vi "ActionVIOnLoad.vi"(8 "error in (no error)":errorcluster, 11 "Device Item Ref in":T1 format="%.0x") -> (0 "error out":errorcluster, 3 "Device Item Ref out":T1 format="%.0x")   [LabVIEW 2019, in "J1939 Addon System Explorer.lvlib"]
uses:
  J1939 Addon System Explorer.lvlib
  <vilib>/NI VeriStand/Custom Device API/Custom Device Item Ref.ctl
  <vilib>/NI VeriStand/Custom Device API/Custom Device Channel.ctl
  <vilib>/NI VeriStand/Custom Device API/Custom Device Channel Type.ctl
  NationalInstruments.VeriStand.SystemDefinitionAPI
  Addon Shared/SubVIs/Constants.vi
  <vilib>/NI/NI VeriStand Advanced SysDef API/_SubVIs/SysDef.Search.GUIDs.vi
  <vilib>/NI/NI VeriStand Advanced SysDef API/_SubVIs/SysDef.Search.Parent.vi
  Addon Shared/J1939 Addon Shared.lvlib
  <vilib>/NI/NI VeriStand Advanced SysDef API/SysDef API/Advanced System Definition.lvlib
  <vilib>/NI VeriStand/Custom Device API/Custom Device API.lvlib
  SubModules/Frame-Protection-Support/Source/System Explorer/Protection and Counter Support System Explorer.lvlib
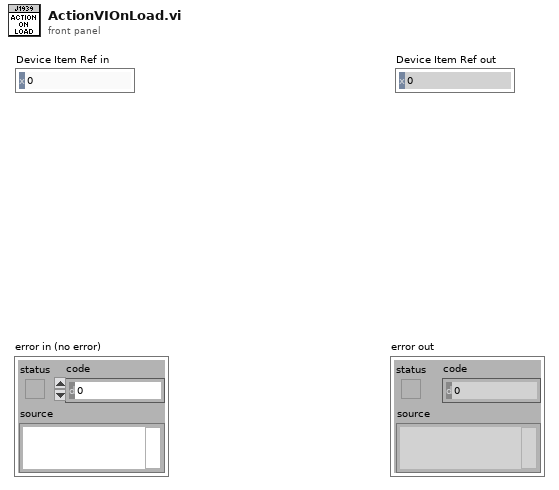
[diagram p1: front panel]
types:
  T1 = typedef "Custom Device API.lvlib/Custom Device Item Ref.ctl" = u64
  T2 = typedef "Custom Device API.lvlib/Custom Device Channel.ctl" = cluster{"Type":T3, "Units":string, "Default Value":dbl, "Faultable":bool, "Scalable":bool}
  T3 = typedef "Custom Device API.lvlib/Custom Device Channel Type.ctl" = enum16{"Input", "Output"}
  T4 = typedef "Protection and Counter Support System Explorer.lvlib/Protection Signal Settings.ctl" = cluster{"Input Channels":T5[], "Protection Type":T6}
  T5 = typedef "Protection and Counter Support System Explorer.lvlib/Protection Signal Linked Channel.ctl" = cluster{"Node Ref":T1}
  T6 = typedef "Protection and Counter Support Shared.lvlib/Protection Type.ctl" = enum16{"Arb ID + Bytes Checksum with Inversion", "Arb ID + Bytes CRC with Inversion", "Reversed Raw Signal Checksum with Inversion", "Concatenated Two's Compliment"}
  T7 = typedef "Advanced System Definition.lvlib/TreeItem.Info.ctl" = cluster{"Name":string, "Description":string, "GUID":string, "Is Channel":bool, "Channel":T2, "Is Waveform":bool, "Waveform":T8}
  T8 = typedef "Custom Device API.lvlib/Custom Device Waveform.ctl" = cluster{"Data Type":T9, "Units":string}
  T9 = typedef "Custom Device API.lvlib/Custom Device Waveform DataType.ctl" = enum16{"Double", "Complex Double"}
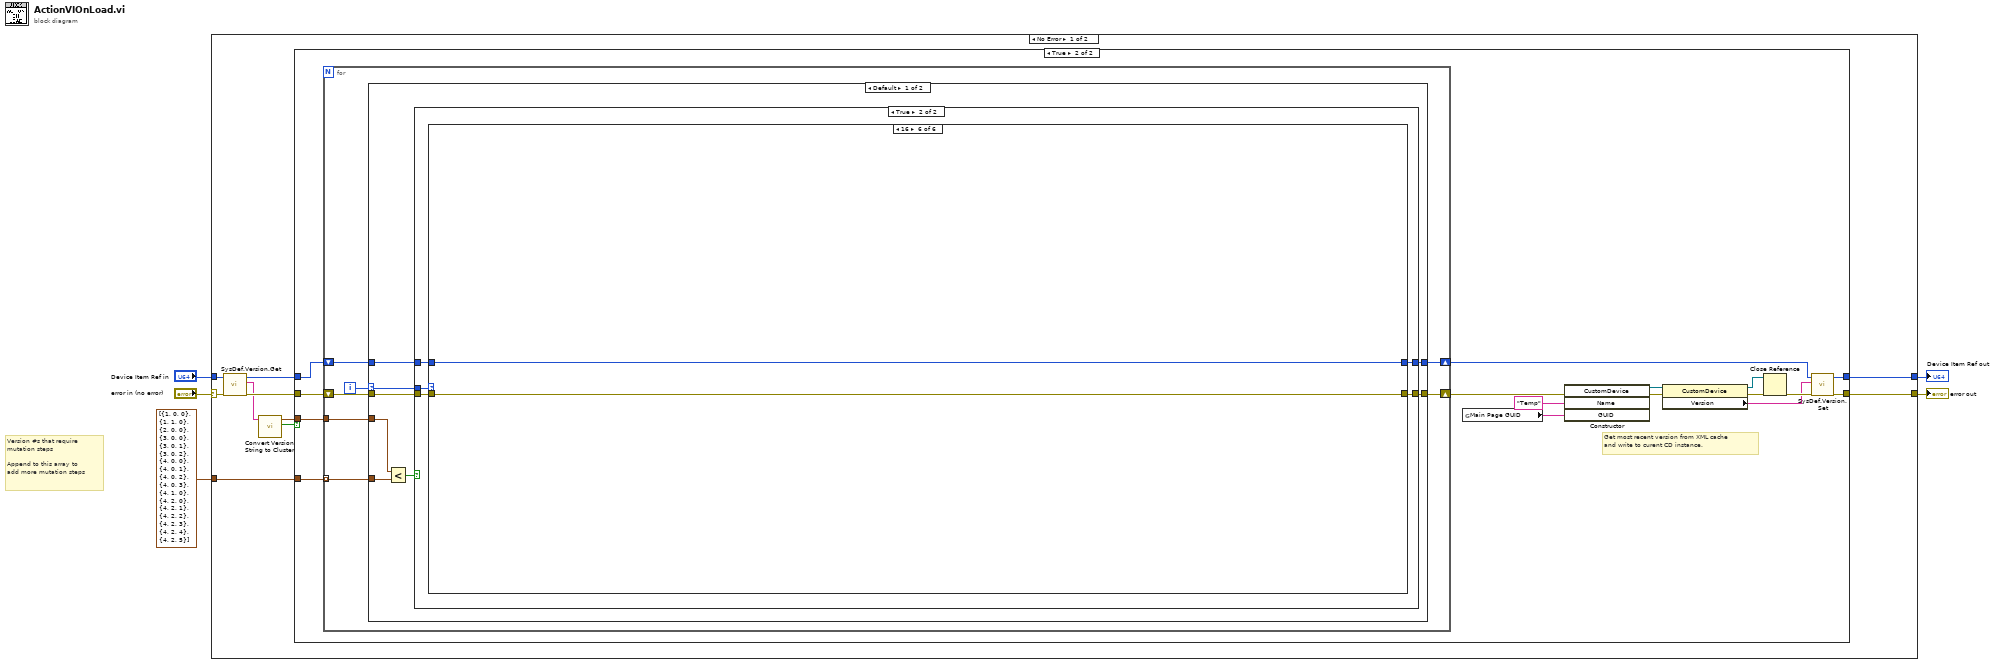
[diagram p0: block diagram]
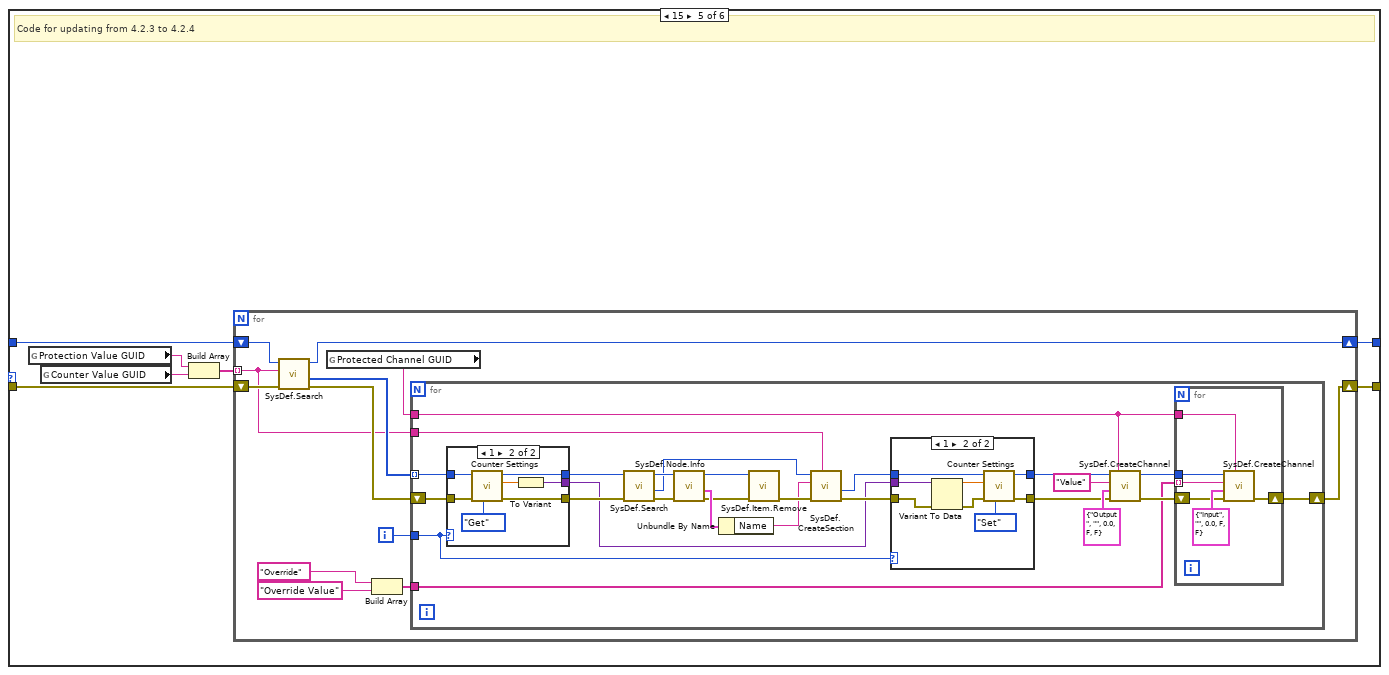
[diagram p8: hidden frame]
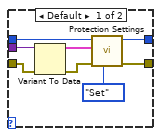
[diagram p9: hidden frame]
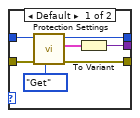
[diagram p10: hidden frame]
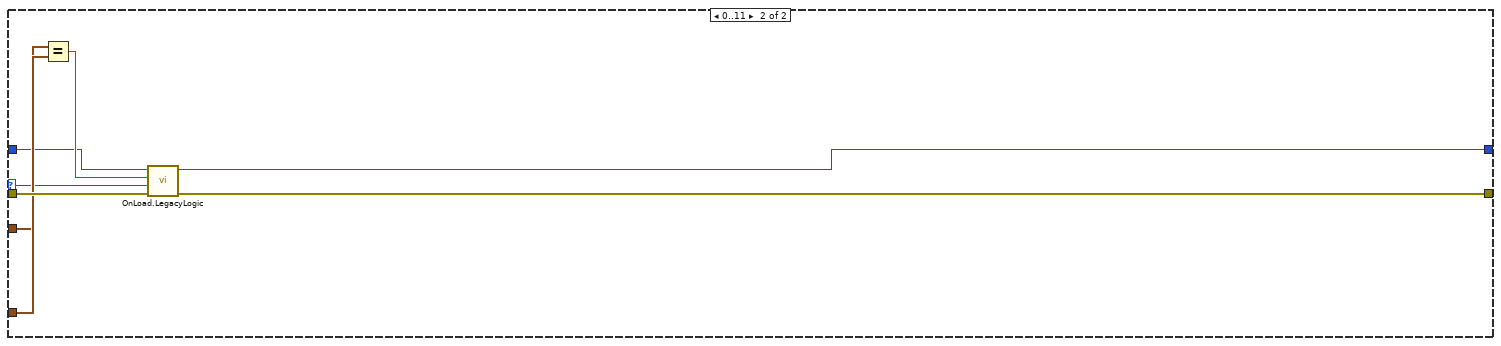
[diagram p11: hidden frame]
diagram:
  # "Version #s that require\nmutation steps\n\nAppend to this array to\nadd more mutation steps"
  n1 = case shown="No Error" "error in (no error)" {
    selector: "error in (no error)" -> [w12 w156]
    tunnel: [w14 w156] -> w1
    tunnel: "Device Item Ref in" -> [w11 w155]
    tunnel: [w13 w155] -> w2
    tunnel: cluster{i32, i32, i32}[] [{1, 0, 0}, {1, 1, 0}, {2, 0, 0}, {3, 0, 0}, {3, 0, 1}, {3, 0, 2}, {4, 0, 0}, {4, 0, 1}, {4, 0, 2}, {4, 0, 3}, {4, 1, 0}, {4, 2, 0}, {4, 2, 1}, {4, 2, 2}, {4, 2, 3}, {4, 2, 4}, {4, 2, 5}] -> [w15 _]
    frame No Error {
      n2 = call <vilib>:"SysDef.Version.Get.vi"("error in (no error)"=w12, "nodeID"=w11) -> ("error out"=w10:errorcluster, "Version"=w8:string, "nodeID out"=w9:u64)  [unwired: 7 in]
      n3 = call "Convert Version String to Cluster.vi"("Version"=w8) -> ("Version Valid?"=w6:bool, "Version"=w7:cluster{i32, i32, i32})  [unwired: 9 in]
      n4 = case shown="True" w6 {
        tunnel: w15 -> [_ w33]
        tunnel: [w17 w26] -> w14
        tunnel: [w16 w25] -> w13
        tunnel: w10 -> [w17 w22]
        tunnel: w9 -> [w16 w21]
        tunnel: w7 -> [_ w18]
        frame False {
        }
        frame True {
          # "Get most recent version from XML cache\nand write to curent CD instance."
          n5 = for {
            tunnel: w33 -> [w40] mode=indexing
            tunnel: w18 -> [w37]
            shift-right: [w35] -> w20
            shift-left: w21 -> [w36]
            shift-right: [w34] -> w19
            shift-left: w22 -> [w38]
            i -> [w39]
            n6 = case shown="Default" w39 {
              selector: w39 -> [w46 w149]
              tunnel: w38 -> [w44 w154]
              tunnel: [w42 w153] -> w34
              tunnel: w36 -> [w43 w147]
              tunnel: [w41 w152] -> w35
              tunnel: w40 -> [w48 w151]
              tunnel: w37 -> [w47 w150]
              frame Default {
                n7 = Less?(x=w47, y=w48) -> (x < y?=w45:bool)
                n8 = case shown="True" w45 {
                  tunnel: w46 -> [_ w55]
                  tunnel: w44 -> [w50 w54]
                  tunnel: w43 -> [w49 w53]
                  tunnel: [w50 w52] -> w42
                  tunnel: [w49 w51] -> w41
                  frame False {
                  }
                  frame True {
                    n9 = case shown="16" w55 {
                      tunnel: w54 -> [w57 w59 w61 w63 w69 w146]
                      tunnel: w53 -> [w56 w58 w60 w62 w66 w145]
                      tunnel: [w57 w59 w61 w63 w68 w146] -> w52
                      tunnel: [w56 w58 w60 w62 w67 w145] -> w51
                      frame 0..11, Default {
                        # "Previous on load scheme. Ignore."
                      }
                      frame 12 {
                        # "Code for updating from 4.2.0 to 4.2.1"
                      }
                      frame 13 {
                        # "Code for updating from 4.2.1 to 4.2.2"
                      }
                      frame 14 {
                        # "Code for updating from 4.2.2 to 4.2.3"
                      }
                      frame 15 {
                        # "Code for updating from 4.2.3 to 4.2.4"
                        n10 = global read "Constants.vi" "Protection Value GUID"() -> (w64:string)
                        n11 = global read "Constants.vi" "Counter Value GUID"() -> (w65:string)
                        n12 = Build Array(w64, w65) -> (w70:string[])
                        n13 = for {
                          shift-right: [w82] -> w67
                          shift-left: w66 -> [w81]
                          shift-right: [w77] -> w68
                          shift-left: w69 -> [w80]
                          tunnel: w70 -> [w73] mode=indexing
                          i -> [w72]
                          n14 = call-poly <vilib>:"SysDef.Search.vi"("error in (no error)"=w80, "GUID"=w73, "nodeID"=w81) -> ("error out"=w78:errorcluster, "Values Out"=w79:u64[], "nodeID out"=w82:u64)  [unwired: 5 in, 1 out]
                          n15 = global read "Constants.vi" "Protected Channel GUID"() -> (w71:string)
                          n16 = Build Array("Override" ("Override Name"), "Override Value" ("Override Value Name")) -> (w74:string[])
                          n17 = for {
                            tunnel: w79 -> [w89] mode=indexing
                            shift-right: [w106] -> w77
                            shift-left: w78 -> [w92]
                            tunnel: w74 -> [w105]
                            tunnel: w71 -> [w103]
                            tunnel: w73 -> [w96]
                            tunnel: w72 -> [w83]
                            n18 = case shown="1" w83 {
                              tunnel: w92 -> [w129 w137]
                              tunnel: [w128 w136] -> w91
                              tunnel: [w127 w135] -> w90
                              tunnel: w89 -> [w130 w134]
                              tunnel: [w125 w132] -> w84
                              frame Default {
                                n19 = call "Protection Settings.vi"("Action"=enum8{"Get", "Set"}."Get", "error in"=w129, "Parent Ref"=w130) -> ("error out"=w128:errorcluster, "Selected Channels"=w126:T4, "Parent Ref Out"=w127:T1)  [unwired: 6 in]
                                n20 = To Variant(anything=w126) -> (Variant=w125:variant)
                              }
                              frame 1 {
                                n21 = call "Counter Settings.vi"("Action"=enum8{"Get", "Set"}."Get", "error in"=w137, "Parent Ref"=w134) -> ("error out"=w136:errorcluster, "Max Count"=w133:dbl, "Parent Ref Out"=w135:T1)  [unwired: 6 in]
                                n22 = To Variant(anything=w133) -> (Variant=w132:variant)
                              }
                            }
                            n23 = call-poly <vilib>:"SysDef.Search.vi"("error in (no error)"=w91, "nodeID"=w90) -> ("error out"=w95:errorcluster, "Value out"=w93:u64, "nodeID out"=w94:u64)  [unwired: 6 in, 1 out]
                            n24 = call <vilib>:"SysDef.Node.Info.vi"("error in (no error)"=w95, "nodeID"=w94) -> ("error out"=w99:errorcluster, "Item Info"=w101:T7, "nodeID out"=w100:u64)  [unwired: 6 in, 1 out]
                            n25 = Unbundle By Name(w101) -> ("Name"=w97:string)
                            n26 = call <vilib>:"SysDef.Item.Remove.vi"("error in (no error)"=w99, "nodeID"=w100) -> ("error out"=w98:errorcluster)  [unwired: 8 in, 1 out]
                            n27 = call <vilib>:"SysDef.CreateSection.vi"("GUID"=w96, "error in (no error)"=w98, "Name"=w97, "nodeID"=w93) -> ("error out"=w88:errorcluster, "New NodeID"=w86:u64)  [unwired: 4 in, 2 out]
                            n28 = case shown="1" w83 {
                              tunnel: w88 -> [w110 w118]
                              tunnel: [w113 w123] -> w87
                              tunnel: w86 -> [w115 w122]
                              tunnel: [w114 w121] -> w85
                              tunnel: w84 -> [w112 w120]
                              frame Default {
                                n29 = Variant To Data(error in=w110, Variant=w112) -> (data=w109:T4, error out=w111:errorcluster)  [unwired: 1 in]
                                n30 = call "Protection Settings.vi"("Action"=enum8{"Get", "Set"}."Set", "error in"=w111, "Selected Channels"=w109, "Parent Ref"=w115) -> ("error out"=w113:errorcluster, "Parent Ref Out"=w114:T1)  [unwired: 5 in, 1 out]
                              }
                              frame 1 {
                                n31 = Variant To Data(error in=w118, Variant=w120) -> (data=w117:dbl, error out=w119:errorcluster)  [unwired: 1 in]
                                n32 = call "Counter Settings.vi"("Action"=enum8{"Get", "Set"}."Set", "error in"=w119, "Max Count"=w117, "Parent Ref"=w122) -> ("error out"=w123:errorcluster, "Parent Ref Out"=w121:T1)  [unwired: 5 in, 1 out]
                              }
                            }
                            n33 = call <vilib>:"SysDef.CreateChannel.vi"("GUID"=w103, "error in (no error)"=w87, "Channel"=T2 {"Type"=enum."Output", "Units"="", "Default Value"=0.0, "Faultable"=FALSE, "Scalable"=FALSE}, "Name"="Value" ("Override Name"), "nodeID"=w85) -> ("error out"=w107:errorcluster, "nodeID out"=w104:u64)  [unwired: 3 in, 2 out]
                            n34 = for {
                              tunnel: w105 -> [w141] mode=indexing
                              tunnel: w104 -> [w140]
                              tunnel: w103 -> [w139]
                              shift-right: [w142] -> w106
                              shift-left: w107 -> [w143]
                              n35 = call <vilib>:"SysDef.CreateChannel.vi"("GUID"=w139, "error in (no error)"=w143, "Channel"=T2 {"Type"=enum."Input", "Units"="", "Default Value"=0.0, "Faultable"=FALSE, "Scalable"=FALSE}, "Name"=w141, "nodeID"=w140) -> ("error out"=w142:errorcluster)  [unwired: 3 in, 3 out]
                            }
                          }
                        }
                      }
                      frame 16 {
                      }
                    }
                  }
                }
              }
              frame 0..11 {
                n36 = Equal?(x=w150, y=w151) -> (x = y?=w148:bool)
                n37 = call "OnLoad.LegacyLogic.vi"("error in (no error)"=w154, "Version Iteration"=w149, "Execute?"=w148, "Device Ref in"=w147) -> ("error out"=w153:errorcluster, "Device Ref out"=w152:T1)  [unwired: 6 in]
              }
            }
          }
          n38 = global read "Constants.vi" "Main Page GUID"() -> (w23:string)
          n39 = constructor class="CustomDevice"(error in=w19, "Name"="Temp", "GUID"=w23) -> (reference out=w32:refnum<k24>, error out=w31:errorcluster)  [unwired: 2 in, 3 out]
          n40 = property class="CustomDevice"(reference=w32, error in=w31) -> (reference out=w29:refnum<k24>, error out=w30:errorcluster, "Version"=w27:string)
          n41 = Close Reference(reference=w29, error in (no error)=w30) -> (error out=w28:errorcluster)
          n42 = call <vilib>:"SysDef.Version.Set.vi"("error in (no error)"=w28, "Version"=w27, "nodeID"=w20) -> ("error out"=w26:errorcluster, "nodeID out"=w25:u64)  [unwired: 7 in]
        }
      }
    }
    frame Error {
    }
  }
  "error out" <- w1
  "Device Item Ref out" <- w2
